vi "niRFUtil MT UTIL Kaiser FIR Filter Design.vi"(2 "Stop Attenuation":dbl format="%.2f", 3 "sampling freq: fs":dbl=1.0 format="%.2f", 4 "high cutoff freq: fh":dbl=0.45 format="%.2f", 5 "low cutoff freq: fl":dbl=0.125 format="%.2f") -> (0 "Estimated Taps":i32, 1 "h":dbl[](array[numeric]) format="%.2f")   [LabVIEW 2015, in "niRFUtil.lvlib"]
uses:
  niRFUtil.lvlib
  <vilib>/Analysis/4window.llb/windowTd.ctl
  <vilib>/Analysis/NI_AALBase.lvlib
  <vilib>/Analysis/NI_AALPro.lvlib
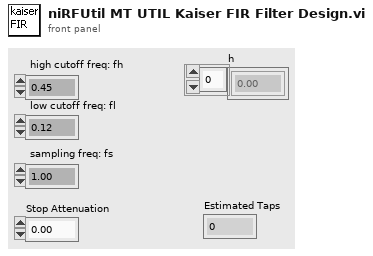
[diagram p1: front panel]
types:
  T1 = typedef "NI_AALPro.lvlib/windowTd.ctl" = u32
  T2 = enum32{"Lowpass", "Highpass", "Bandpass", "Bandstop"}
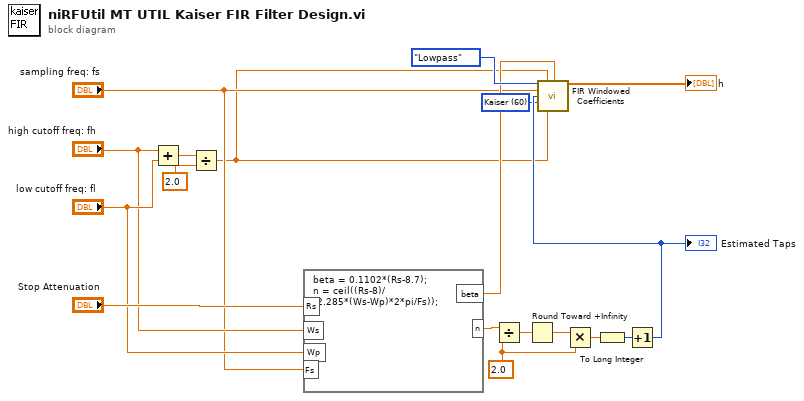
[diagram p0: block diagram]
diagram:
  w3 = T1 60 items=["Rectangle"=0, "Hanning"=1, "Hamming"=2, "Blackman-Harris"=3, "Exact Blackman"=4, "Blackman"=5, "Flat Top"=6, "4 Term B-Harris "=7, "7 Term B-Harris"=8, "Low Sidelobe"=9, "Blackman Nuttall"=11, "Triangle"=30, "Bartlett-Hanning"=31, "Bohman"=32, "Parzen"=33, "Welch"=34, "Kaiser"=60, "Dolph-Chebyshev"=61, "Gaussian"=62] ("window")
  w12 = 2.0 ("y")
  n1 = Add(x="high cutoff freq: fh", y="low cutoff freq: fl") -> (x+y=w18:dbl)
  n2 = Divide(x=w18, y=2.0) -> (x/y=w1:dbl)
  n3 = formula code="beta = 0.1102*(Rs-8.7);\nn = ceil((Rs-8)/(2.285*(Ws-Wp)*2*pi/Fs));"("Rs"="Stop Attenuation", "Ws"="high cutoff freq: fh", "Wp"="low cutoff freq: fl", "Fs"="sampling freq: fs") -> ("beta"=w4:dbl, "n"=w13:dbl)
  n4 = Divide(x=w13, y=w12) -> (x/y=w9:dbl)
  n5 = Round Toward +Infinity(x=w9) -> (ceil(x): smallest int >= x=w8:dbl)
  n6 = Multiply(x=w8, y=w12) -> (x*y=w11:dbl)
  n7 = To Long Integer(number=w11) -> (32bit integer=w10:i32)
  n8 = Increment(x=w10) -> (x+1=w5:i32)
  "Estimated Taps" <- w5
  n9 = call <vilib>:"FIR Windowed Coefficients.vi"("filter type"=T2."Lowpass", "high cutoff freq: fh"=w1, "window parameter"=w4, "sampling freq: fs"="sampling freq: fs", "taps"=w5, "window"=w3, "low cutoff freq: fl"=w1) -> ("FIR Windowed Coefficients"=→"h":dbl[])  [unwired: 7 in, 1 out]
